vi "Step In.vi"(8 "error in (no error)":errorcluster, 9 "elements":cluster{"State":string, "Data":variant}[](array[cluster]), 10 "?":T1, 11 "QUEUE in":refnum<queue>) -> (0 "error out":errorcluster, 3 "queue out":refnum<queue>)   [LabVIEW 2016]
uses:
  QueueAct.ctl
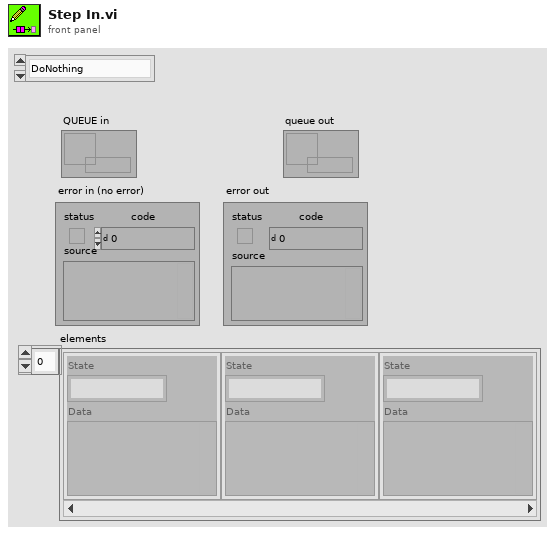
[diagram p1: front panel]
types:
  T1 = typedef "QueueAct.ctl" = enum16{"DoNothing", "AddAfter", "AddBefore", "DeleteOne", "Clear"}
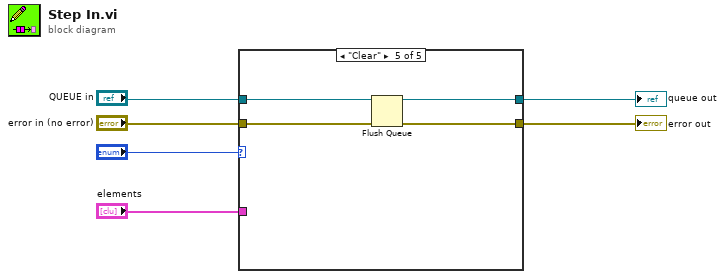
[diagram p0: block diagram]
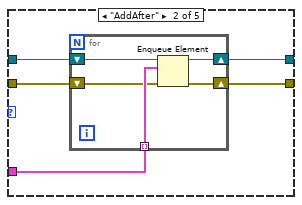
[diagram p3: hidden frame]
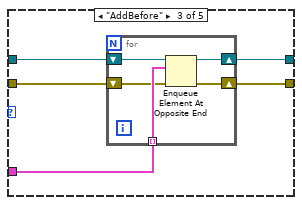
[diagram p4: hidden frame]
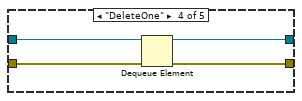
[diagram p5: hidden frame]
diagram:
  n1 = case shown="\"Clear\"" "?" {
    tunnel: [w8 w13 w23 w32 w35] -> w2
    tunnel: [w7 w12 w22 w31 w33] -> w1
    tunnel: "elements" -> [_ w11 w21 _ _]
    tunnel: "QUEUE in" -> [w8 w10 w20 w30 w36]
    tunnel: "error in (no error)" -> [w7 w9 w19 w29 w34]
    frame "DoNothing", Default {
    }
    frame "AddAfter" {
      n2 = for {
        tunnel: w11 -> [w16] mode=indexing
        shift-right: [w18] -> w13
        shift-left: w10 -> [w15]
        shift-right: [w17] -> w12
        shift-left: w9 -> [w14]
        n3 = Enqueue Element(queue=w15, element=w16, error in (no error)=w14) -> (queue out=w18:refnum<queue>, error out=w17:errorcluster)  [unwired: 1 in, 1 out]
      }
    }
    frame "AddBefore" {
      n4 = for {
        tunnel: w21 -> [w26] mode=indexing
        shift-right: [w28] -> w23
        shift-left: w20 -> [w25]
        shift-right: [w27] -> w22
        shift-left: w19 -> [w24]
        n5 = Enqueue Element At Opposite End(queue=w25, element=w26, error in (no error)=w24) -> (queue out=w28:refnum<queue>, error out=w27:errorcluster)  [unwired: 1 in, 1 out]
      }
    }
    frame "DeleteOne" {
      n6 = Dequeue Element(queue=w30, error in (no error)=w29) -> (queue out=w32:refnum<queue>, error out=w31:errorcluster)  [unwired: 1 in, 2 out]
    }
    frame "Clear" {
      n7 = Flush Queue(queue=w36, error in (no error)=w34) -> (queue out=w35:refnum<queue>, error out=w33:errorcluster)  [unwired: 1 out]
    }
  }
  "error out" <- w1
  "queue out" <- w2
